vi "SLSC Add Item to Tree with Properties.vi"(6 "Child Text":string[](array[string]), 8 "Glyph Index":i32, 9 "Item indent":i32, 10 "Child Tag":string, 11 "Left Cell String":string) -> (3 "Item":T1)   [LabVIEW 2017, in "SLSC Tree Control.lvlib"]
doc: "Create Item from elements to the Tree Control."
uses:
  SLSC Tree Control.lvlib
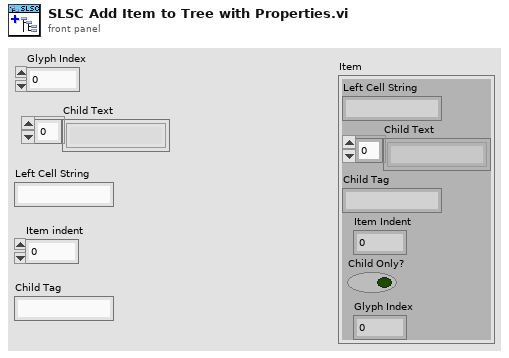
[diagram p1: front panel]
types:
  T1 = cluster{"Left Cell String":string, "Child Text":string[], "Child Tag":string, "Item Indent":i32, "Child Only?":bool, "Glyph Index":i32}
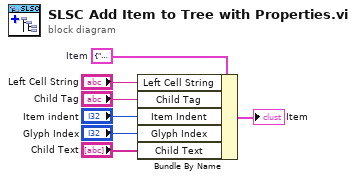
[diagram p0: block diagram]
diagram:
  w4 = T1 {"Left Cell String"="", "Child Text"=[], "Child Tag"="", "Item Indent"=0, "Child Only?"=FALSE, "Glyph Index"=0}  # Item
  n1 = Bundle By Name(cluster=w4, "Left Cell String"="Left Cell String", "Child Tag"="Child Tag", "Item Indent"="Item indent", "Glyph Index"="Glyph Index", "Child Text"="Child Text") -> (→"Item":T1)
